vi "TDMS Advanced Basic Asynchronous Read.vi"() -> ()   [LabVIEW 2023]
doc: "This example demonstrates how to read a given number or all of the data samples asynchronously from a .tdms file using the Advanced TDMS functions."
panel:
  out "Waveform Graph":u32[](graph)
  # "Overview: Demonstrates how to read a given number or all of the data samples asynchronously from a .tdms file using the Advanced TDMS functions.\nInstructions:\n1. Make sure you have already run TDMS Advanced Asynchronous Write.vi.\n2. Run the VI.\n3. Delete the TDMS file (located at [LabVIEW Data]\\Example TDMS Advanced Asynchronous Write.tdms) when you are done."
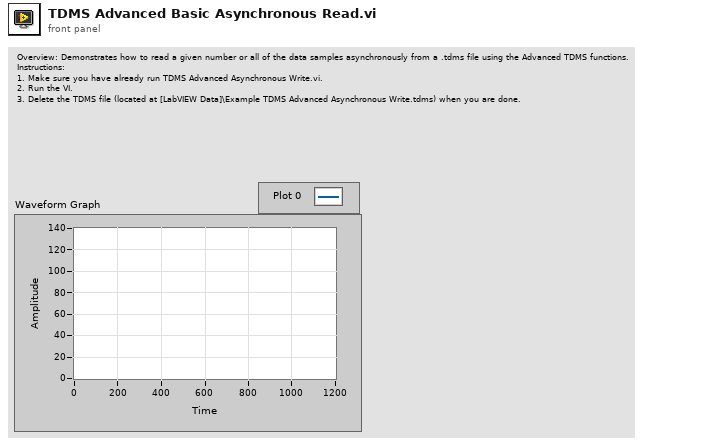
[diagram p1: front panel]
types:
  T1 = enum16{"open", "open or create", "create or replace", "create", "open (read-only)"}
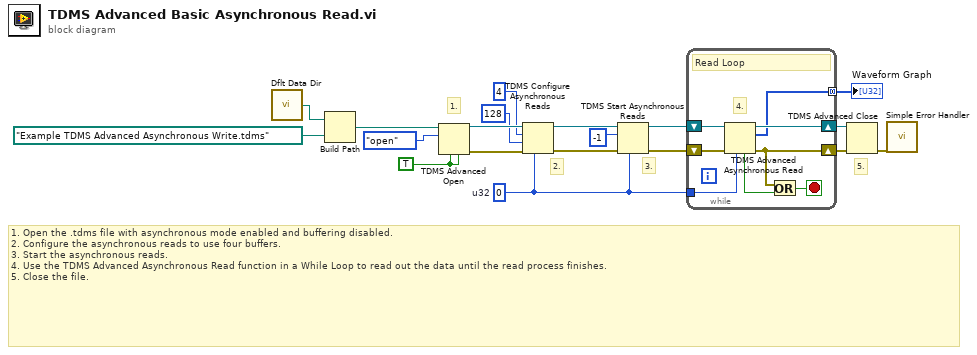
[diagram p0: block diagram]
diagram:
  w5 = u32 0  # u32
  w15 = TRUE ("enable asynchronous? (T)")
  # "3."
  # "2."
  # "1. Open the .tdms file with asynchronous mode enabled and buffering disabled.\n2. Configure the asynchronous reads to use four buffers.\n3. Start the asynchronous reads.\n4. Use the TDMS Advanced Asynchronous Read function in a While Loop to read out the data until the read process finishes.\n5. Close the file."
  # "1."
  # "5."
  n1 = call <vilib>:"Dflt Data Dir.vi"() -> ("App:Default Data Directory"=w16:path)
  n2 = Build Path(base path=w16, name or relative path=path "Example TDMS Advanced Asynchronous Write.tdms") -> (appended path=w18:path)
  n3 = TDMS Advanced Open(4:w15, 6:w15, 10:T1."open" ("operation (0:open)"), 11:w18) -> (0:w13:errorcluster, 3:w14:refnum<k34>)  [unwired: 1 in, 1 out]
  n4 = TDMS Configure Asynchronous Reads(6:w5, 8:w13, 9:u32 128 ("buffer size"), 10:u32 4 ("number of buffers (4)"), 11:w14) -> (0:w9:errorcluster, 3:w10:refnum<k34>)  [unwired: 1 in]
  n5 = TDMS Start Asynchronous Reads(6:w5, 8:w9, 10:i64 -1 ("total count (-1)"), 11:w10) -> (0:w6:errorcluster, 3:w7:refnum<k34>)
  n6 = while {
    shift-right: [w25] -> w3
    shift-left: w7 -> [w27]
    shift-right: [w21] -> w4
    shift-left: w6 -> [w26]
    tunnel: w5 -> [w24]
    tunnel: [w20] -> w1 mode=concatenating
    stop <- w23 stop-if-true
    # "4."
    # "Read Loop"
    n7 = TDMS Advanced Asynchronous Read(6:w24, 8:w26, 11:w27) -> (0:w21:errorcluster, 2:w20:u32[], 3:w25:refnum<k34>, 4:w22:bool)
    n8 = Or(x=w21, y=w22) -> (x .or. y?=w23:bool)
  }
  "Waveform Graph" <- w1
  n9 = TDMS Advanced Close(8:w4, 11:w3) -> (0:w2:errorcluster)  [unwired: 2 in, 1 out]
  n10 = call <vilib>:"Simple Error Handler.vi"("error in (no error)"=w2) -> ()  [unwired: 4 in, 5 out]
